vi "DIO_PWM.vi"(0 "DIO.OUT":bool, 1 "DIO.DIR":bool, 2 "PWM.CS":u8, 3 "PWM.CNFG":u8 format="%08b", 4 "PWM.CMP":u16, 5 "PWM.MAX":u16, 6 "DIO/PWM":refnum<k21>, 7 "SELECT":bool) -> (14 "DIO.IN":bool, 19 "PWM.CNTR":u16)   [LabVIEW 2018]
doc: "This VI switches between the DIO functionality and the PWM functionality for the specified FPGA I/O channels.\n- If <b>SELECT</b> is FALSE, DIO is enabled.\n- If <b>SELECT</b> is TRUE, PWM is enabled."
panel:
  # "This VI switches between the DIO functionality and the PWM functionality for the specified FPGA I/O channels.\n- If SELECT is FALSE, DIO is enabled.\n- If SELECT is TRUE, PWM is enabled."
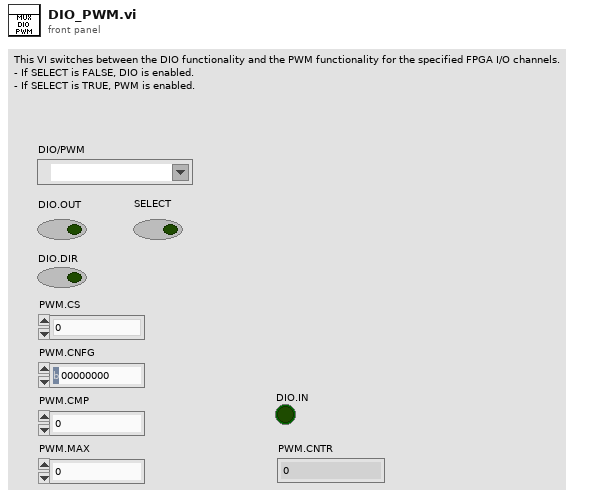
[diagram p1: front panel]
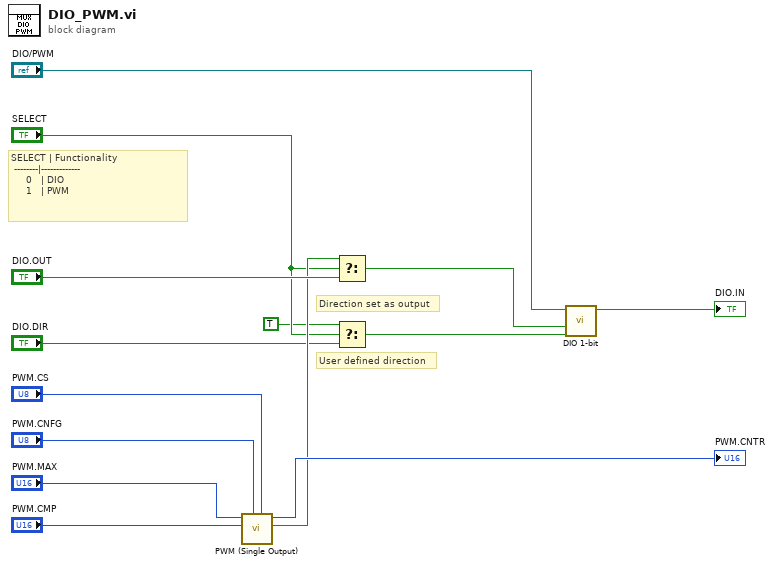
[diagram p0: block diagram]
diagram:
  # "Direction set as output"
  # "User defined direction"
  # "SELECT | Functionality \n --------|-------------\n     0   | DIO\n     1   | PWM"
  n1 = call "PWM (Single Output).vi"("Clock Select"="PWM.CS", "Counter Control"="PWM.CNFG", "Output Compare Value"="PWM.CMP", "Max Counter Value"="PWM.MAX") -> ("Output"=w8:bool, "Counter Value"=→"PWM.CNTR":u16)  [unwired: 6 in]
  n2 = Select(t=w8, s="SELECT", f="DIO.OUT") -> (s? t:f=w10:bool)
  n3 = Select(t=TRUE, s="SELECT", f="DIO.DIR") -> (s? t:f=w4:bool)
  n4 = call "DIO 1-bit.vi"("DIR"=w4, "OUT"=w10, "DIO Refnum"="DIO/PWM") -> ("IN"=→"DIO.IN":bool)  [unwired: 8 in]
